vi "Draw.vi"(8 "error in (no error)":errorcluster, 10 "Snake in 2":refnum<class "SnakeGame.lvclass">, 11 "Snake in":refnum<class "Snake.lvclass">) -> (0 "error out":errorcluster, 2 "Snake out 2":refnum<class "SnakeGame.lvclass">, 3 "Snake out":refnum<class "Snake.lvclass">)   [LabVIEW 2019, in "RT_Game.lvlib" / "Snake.lvclass"]
uses:
  Snake.lvclass
  SnakeGame/SnakeGame.lvclass
  C:/Users/FreshBob/Dropbox/VIs/myRIO_GameConsole/RT/RT_Game/Game/Game.lvclass
  Snake.lvclass/Snake.ctl
  Game/Game.lvclass
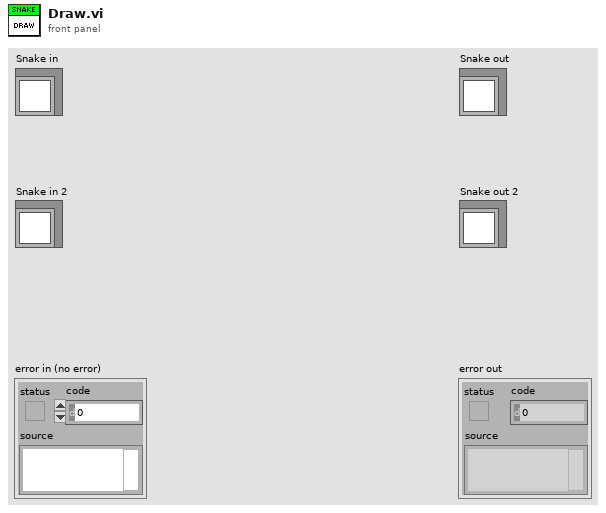
[diagram p1: front panel]
types:
  T1 = typedef "RT_Game.lvlib/SnakeGame.lvclass/CoordinateData.ctl" = cluster{"Coordinate":T2, "TileCode":u16}
  T2 = typedef "RT_Game.lvlib/Game.lvclass/Coordinate.ctl" = cluster{"x":dbl, "y":dbl}
  T3 = typedef "RT_Game.lvlib/SnakeGame.lvclass/Direction.ctl" = enum16{"Up", "Left", "Down", "Right"}
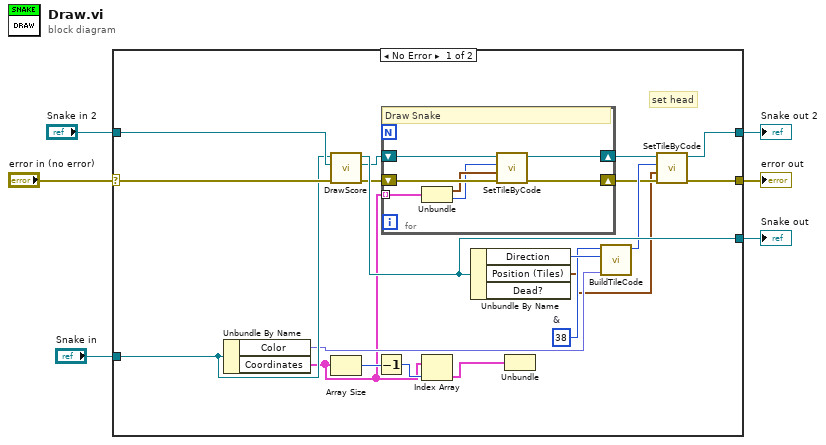
[diagram p0: block diagram]
diagram:
  n1 = case shown="No Error" "error in (no error)" {
    selector: "error in (no error)" -> [w25 w35]
    tunnel: [w24 w35] -> w5
    tunnel: [w20 w34] -> w3
    tunnel: "Snake in" -> [w22 w34]
    tunnel: "Snake in 2" -> [w23 w33]
    tunnel: [w21 w33] -> w1
    frame No Error {
      w16 = u16 38  # &
      # "set head"
      n2 = Unbundle By Name(w22) -> ("Color"=w18:fxp<+,3,3>, "Coordinates"=w12:T1[])
      n3 = call "DrawScore.vi"("error in (no error)"=w25, "Pong in"=w23, "Snake in"=w22) -> ("error out"=w9:errorcluster, "Pong out"=w8:refnum<class "SnakeGame.lvclass">, "Snake out"=w20:refnum<class "Snake.lvclass">)  [unwired: 6 in]
      n4 = Array Size(array=w12) -> (size(s)=w13:i32)
      n5 = Decrement(x=w13) -> (x-1=w14:i32)
      n6 = for {
        shift-right: [w31] -> w11
        shift-left: w9 -> [w32]
        shift-right: [w30] -> w10
        shift-left: w8 -> [w26]
        tunnel: w12 -> [w29] mode=indexing
        # "Draw Snake"
        n7 = Unbundle(w29) -> ("Coordinate"=w28:T2, "TileCode"=w27:u16)
        n8 = call "SetTileByCode.vi"("error in (no error)"=w32, "Coordinates"=w28, "TileNumber"=w27, "Game in"=w26) -> ("error out"=w31:errorcluster, "Game out"=w30:refnum<class "SnakeGame.lvclass">)  [unwired: 6 in]
      }
      n9 = Index Array(array=w12, index=w14) -> (element=w15:T1)
      n10 = Unbundle By Name(w20) -> ("Direction"=w17:T3, "Position (Tiles)"=w7:T2)  [unwired: 1 out]
      n11 = Unbundle(w15) -> ()  [unwired: 2 out]
      n12 = call "BuildTileCode.vi"("replace_color"=w18, "rotation"=w17, "tilenumber"=w16) -> ("TileCode"=w19:u16)  [unwired: 8 in]
      n13 = call "SetTileByCode.vi"("error in (no error)"=w11, "Coordinates"=w7, "TileNumber"=w19, "Game in"=w10) -> ("error out"=w24:errorcluster, "Game out"=w21:refnum<class "SnakeGame.lvclass">)  [unwired: 6 in]
    }
    frame Error {
    }
  }
  "error out" <- w5
  "Snake out" <- w3
  "Snake out 2" <- w1
